vi "Read Averaging time.vi"(8 "error in (no error)":errorcluster, 11 "Write Averaging time Msg in":refnum<class "Write Averaging time Msg.lvclass">) -> (0 "error out":errorcluster, 2 "Averaging time":dbl, 3 "Write Averaging time Msg out":refnum<class "Write Averaging time Msg.lvclass">)   [LabVIEW 2015, in "Write Averaging time Msg.lvclass"]
uses:
  Write Averaging time Msg.lvclass
  Write Averaging time Msg.lvclass/Write Averaging time Msg.ctl
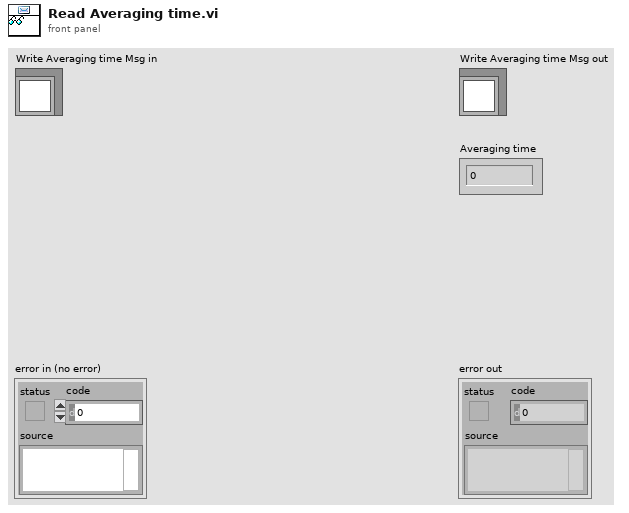
[diagram p1: front panel]
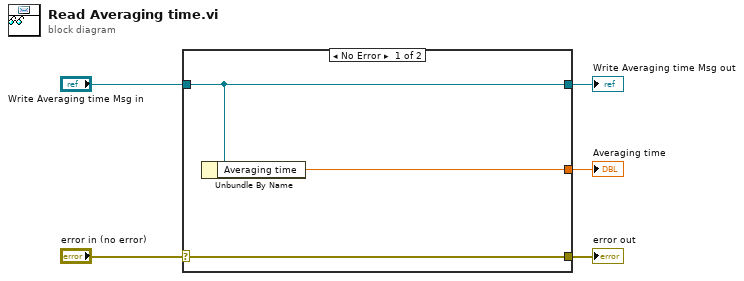
[diagram p0: block diagram]
diagram:
  n1 = case shown="No Error" "error in (no error)" {
    selector: "error in (no error)" -> [w8 w9]
    tunnel: [w8 w9] -> w4
    tunnel: [w7 w10] -> w2
    tunnel: "Write Averaging time Msg in" -> [w7 w10]
    tunnel: [w6 _] -> w1
    frame No Error {
      n2 = Unbundle By Name(w7) -> ("Averaging time"=w6:dbl)
    }
    frame Error {
    }
  }
  "error out" <- w4
  "Write Averaging time Msg out" <- w2
  "Averaging time" <- w1
